vi "Rx.vi"() -> ()   [LabVIEW 2013]
panel:
  in  "VLS Valves":bool=TRUE
  out "TI-603":dbl format="%.1f"
  out "TI-640":dbl format="%.1f"
  out "TI-630":dbl format="%.1f"
  out "TI-622":dbl format="%.1f"
  out "TI-611":dbl format="%.1f"
  out "TI-503":dbl format="%.1f"
  in  "XV-641":bool
  in  "XV-640":bool
  in  "XV-630":bool
  out "FAF1":bool
  out "TI-620":dbl format="%.1f"
  out "TI-502":dbl format="%.1f"
  out "AFE":bool
  out "AFE3":bool
  out "AFE2":bool
  out "AFE1":bool
  out "PI-641":dbl format="%.1f"
  out "TI-641":dbl format="%.1f"
  out "FI-641":dbl format="%.1f"
  out "TI-631":dbl format="%.1f"
  out "PI-621":dbl format="%.1f"
  out "TI-621":dbl format="%.1f"
  out "TI-610":dbl format="%.1f"
  out "AF":bool
  out "V-600 O2":dbl format="%.1f"
  out "TI-602":dbl format="%.1f"
  out "PI-600":dbl format="%.1f"
  out "TI-601":dbl format="%.1f"
  out "TI-600":dbl format="%.1f"
  out "Ash KO 1":bool
  out "Ash KO 3":bool
  out "Ash KO 2":bool
  out "AKOE":bool
  out "1 LO":bool
  out "1 HI":bool
  out "2 LO":bool
  out "2 HI":bool
  out "FAFE":bool
  in  "PCV-641":dbl format="%.2f"
  out "PCV-641 PV":dbl format="%.2f"
  out "AF 1":bool
  out "FAF":bool
  out "Bottom":dbl format="%.3f"
  out "Middle":dbl format="%.3f"
  out "Top":dbl format="%.3f"
  out "TI-500E":dbl format="%.1f"
  out "TI-500C":dbl format="%.1f"
  out "TI-500A":dbl format="%.1f"
  in  "HX-500":bool
  in  "TI-530 2":dbl
  in  "TI-520 2":dbl
  in  "TI-510 2":dbl
  out "TI-530":dbl format="%.1f"
  out "TI-520":dbl format="%.1f"
  out "TI-510":dbl format="%.1f"
  # "Power KVA"
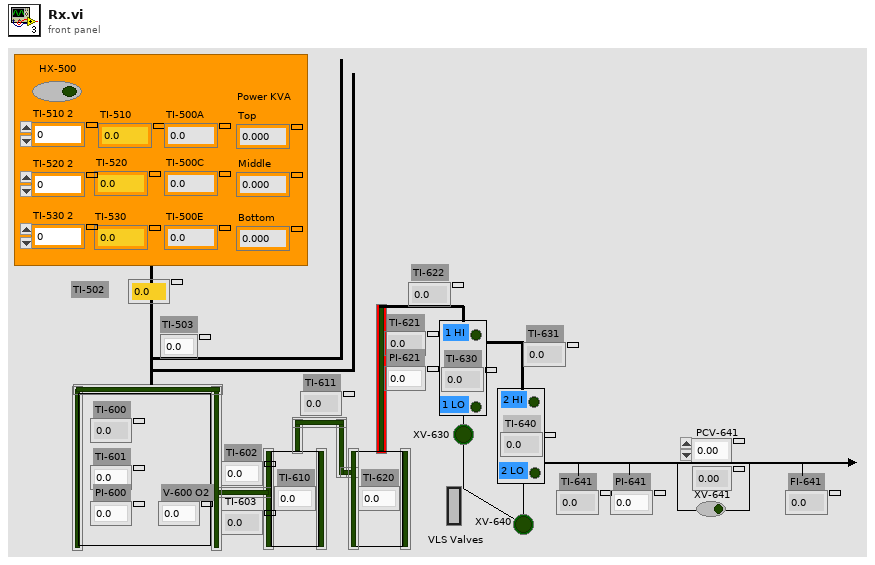
[diagram p1: front panel]
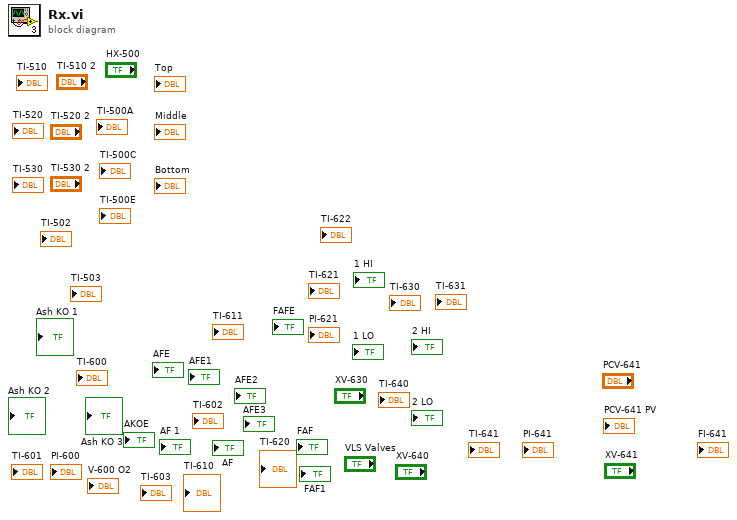
[diagram p0: block diagram]
diagram:
